vi "Read Configuration.vi"(10 "XML File Path conf":path=path "c:/ni-rt/startup/configuration.xml", 11 "Error In":errorcluster) -> (0 "Matrices":T2, 1 "Configuration":T3={"Accelerometer Bias"={"X (m/s)"=0.0, "Y (m/s)"=0.0, "Z (m/s)"=0.0}, "Gyroscope Bias"={"X (m/s)"=0.0, "Y (m/s)"=0.0, "Z (m/s)"=0.0}, "Steering Motor Gear Ratio"=611.0, "Steering Pully Gear Ratio"=1.0, "Steering Encoder CPR"=500.0, "Steering Motor Max RPM"=4000.0, "Wheelbase (m)"=1.12, "Fork Angle (rad)"=1.3, "Balancing Controller"={"Kp (/s)"=0.0, "Kd (1)"=0.0}, "Max Allowed Steering Angle (rad)"=0.7, "Task Periods"={"Emergency Stop (us)"=0, "IMU (us)"=0, "Steering Motor Encoder (us)"=0, "State Estimator (us)"=0, "Balancing Controller (us)"=0, "GNSS (us)"=0, "Logging (us)"=0, "Drive Motor (us)"=0}, "Drive Motor Gear Ratio"=0.7, "lr"=0.0, "lf"=0.0, "lambda"=0.0, "k1"=0.0, "k2"=0.0, "e1_max"=0.0, "Ad_t"=0.0, "Bd_t"=0.0, "C_t"=0.0, "D_t"=0.0, "Wheel radius"=0.311}, 2 "value":T1, 3 "Error Out":errorcluster, 5 "init trajectory 2":dbl[][](array[numeric]))   [LabVIEW 2021]
uses:
  Configuration.ctl
  <vilib>/Analysis/Matrix/Datatypes/RealMatrix.ctl
  <vilib>/Utility/xml.llb/Read From XML File(string).vi
  <vilib>/Analysis/Matrix/Numeric/Conversions/Matrix To Array - RM.vi
  <vilib>/Analysis/Matrix/NI_Matrix.lvlib
panel:
  in  "init trajectory":dbl[][](array[numeric])
  in  "XML File Path traj":path=path "c:/ni-rt/startup/trajectorylab.xml"
  in  "Init Matrix":T1
  in  "XML File Path matr":path=path "c:/ni-rt/startup/matrixlab.xml"
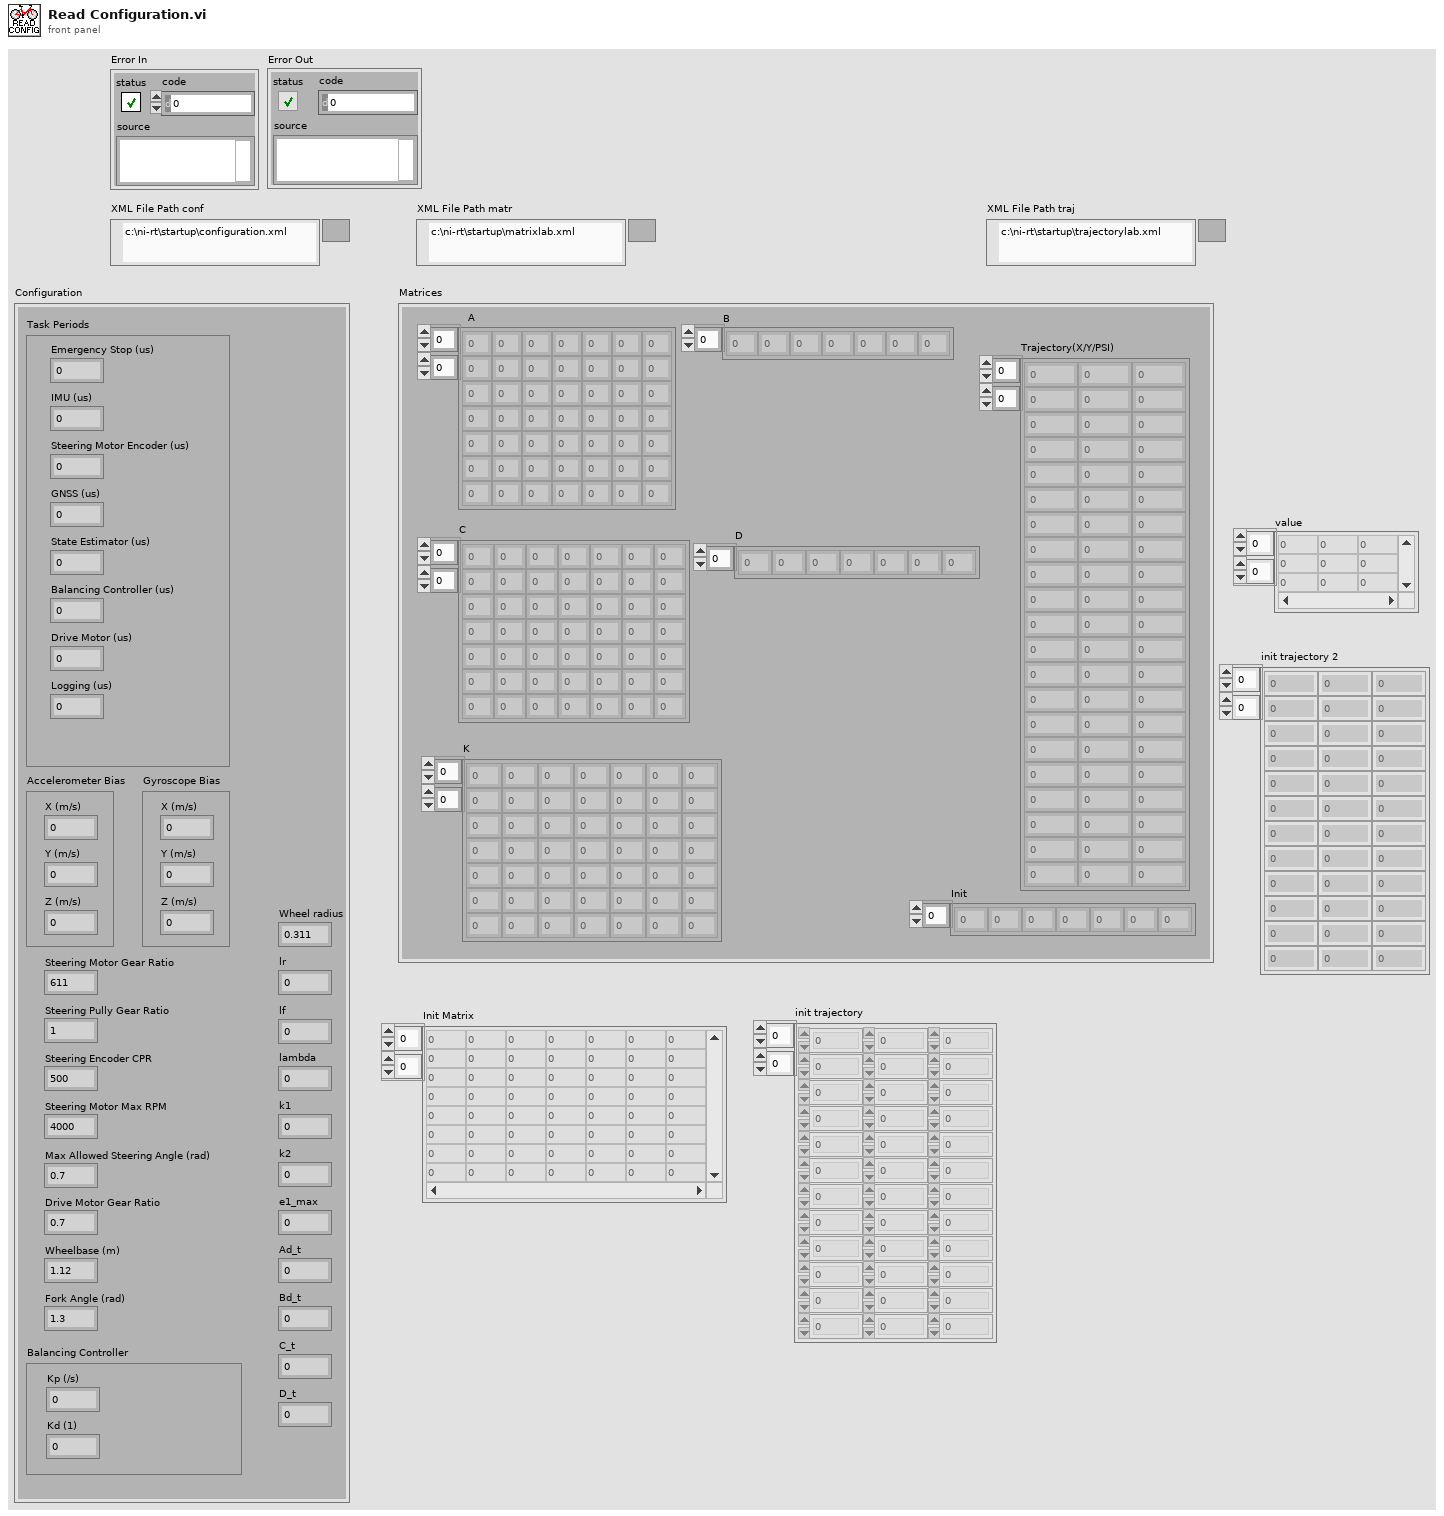
[diagram p1: front panel]
types:
  T1 = typedef "NI_Matrix.lvlib/RealMatrix.ctl" = dbl[][]
  T2 = cluster{"B":dbl[], "A":dbl[][], "C":dbl[][], "D":dbl[], "K":dbl[][], "Trajectory(X/Y/PSI)":dbl[][], "Init":dbl[]}
  T3 = typedef "Configuration.ctl" = cluster{"Accelerometer Bias":cluster{"X (m/s)":dbl, "Y (m/s)":dbl, "Z (m/s)":dbl}, "Gyroscope Bias":cluster{"X (m/s)":dbl, "Y (m/s)":dbl, "Z (m/s)":dbl}, "Steering Motor Gear Ratio":dbl, "Steering Pully Gear Ratio":dbl, "Steering Encoder CPR":dbl, "Steering Motor Max RPM":dbl, "Wheelbase (m)":dbl, "Fork Angle (rad)":dbl, "Balancing Controller":cluster{"Kp (/s)":dbl, "Kd (1)":dbl}, "Max Allowed Steering Angle (rad)":dbl, "Task Periods":cluster{"Emergency Stop (us)":i64, "IMU (us)":i64, "Steering Motor Encoder (us)":i64, "State Estimator (us)":i64, "Balancing Controller (us)":i64, "GNSS (us)":i64, "Logging (us)":i64, "Drive Motor (us)":i64}, "Drive Motor Gear Ratio":dbl, "lr":dbl, "lf":dbl, "lambda":dbl, "k1":dbl, "k2":dbl, "e1_max":dbl, "Ad_t":dbl, "Bd_t":dbl, "C_t":dbl, "D_t":dbl, "Wheel radius":dbl}
  T4 = cluster{"B":dbl[], "A":dbl[][], "C":dbl[][], "D":dbl[], "K":dbl[][], "Trajectory":dbl[][], "Init":dbl[]}
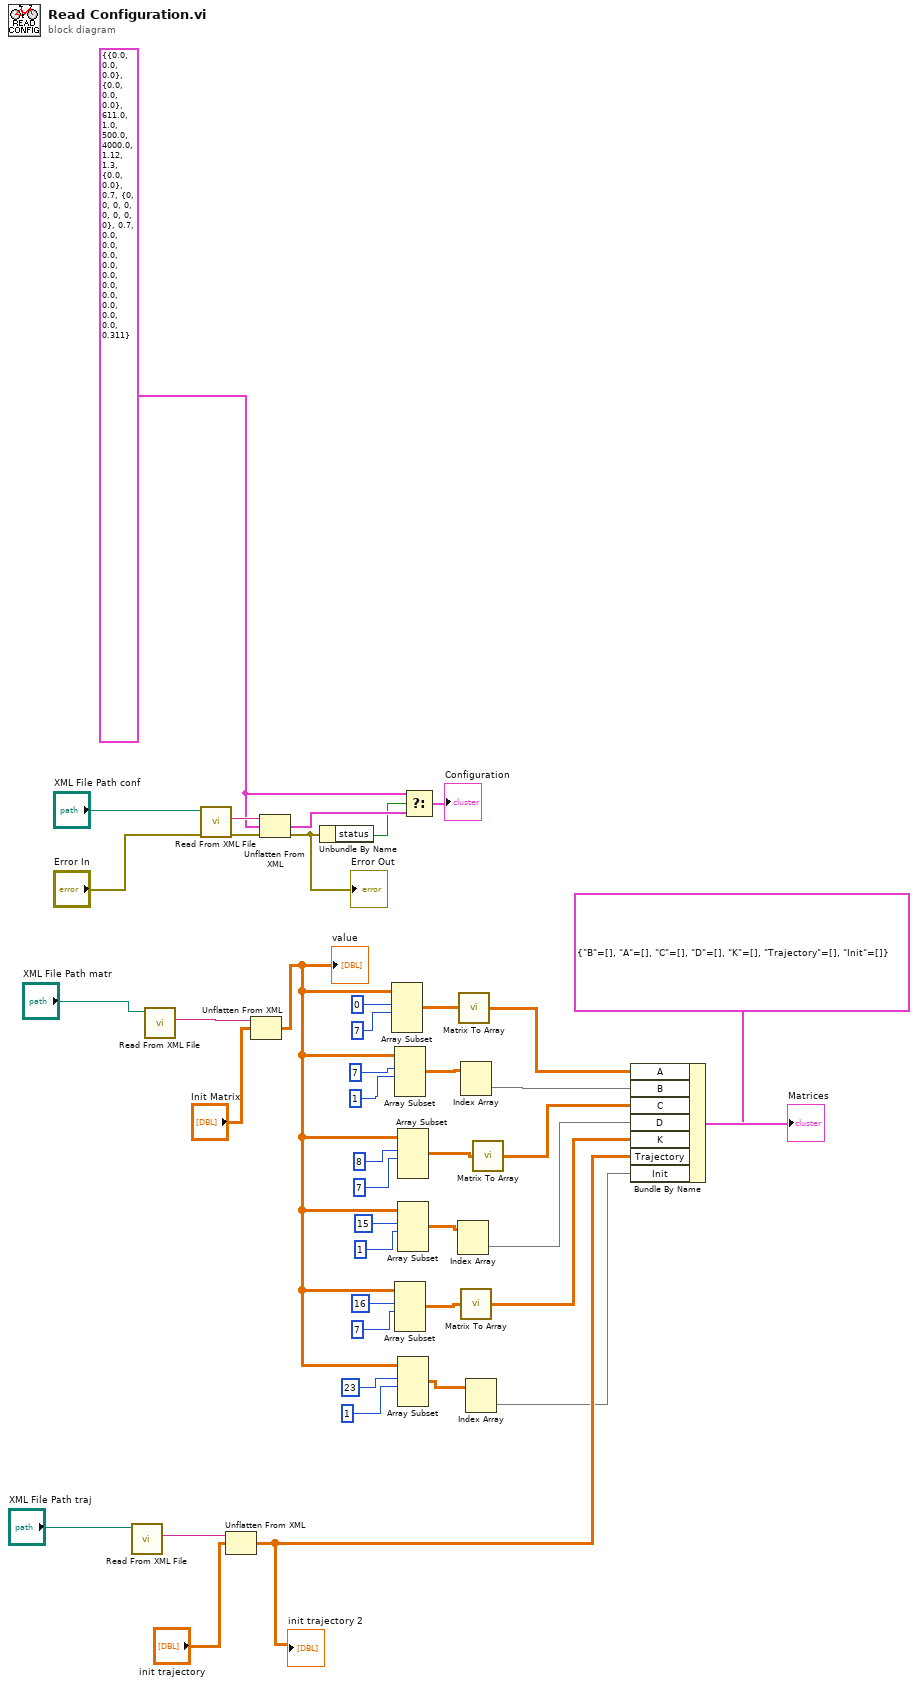
[diagram p0: block diagram]
diagram:
  w38 = T3 {"Accelerometer Bias"={"X (m/s)"=0.0, "Y (m/s)"=0.0, "Z (m/s)"=0.0}, "Gyroscope Bias"={"X (m/s)"=0.0, "Y (m/s)"=0.0, "Z (m/s)"=0.0}, "Steering Motor Gear Ratio"=611.0, "Steering Pully Gear Ratio"=1.0, "Steering Encoder CPR"=500.0, "Steering Motor Max RPM"=4000.0, "Wheelbase (m)"=1.12, "Fork Angle (rad)"=1.3, "Balancing Controller"={"Kp (/s)"=0.0, "Kd (1)"=0.0}, "Max Allowed Steering Angle (rad)"=0.7, "Task Periods"={"Emergency Stop (us)"=0, "IMU (us)"=0, "Steering Motor Encoder (us)"=0, "State Estimator (us)"=0, "Balancing Controller (us)"=0, "GNSS (us)"=0, "Logging (us)"=0, "Drive Motor (us)"=0}, "Drive Motor Gear Ratio"=0.7, "lr"=0.0, "lf"=0.0, "lambda"=0.0, "k1"=0.0, "k2"=0.0, "e1_max"=0.0, "Ad_t"=0.0, "Bd_t"=0.0, "C_t"=0.0, "D_t"=0.0, "Wheel radius"=0.311} ("Configuration")
  n1 = call-poly <vilib>:"Read From XML File.vi"("XML File Path"="XML File Path traj") -> ("XML Elements"=w9:string)  [unwired: 8 in, 2 out]
  n2 = call-poly <vilib>:"Read From XML File.vi"("XML File Path"="XML File Path matr") -> ("XML Elements"=w34:string)  [unwired: 8 in, 2 out]
  n3 = call-poly <vilib>:"Read From XML File.vi"("error in (no error)"="Error In", "XML File Path"="XML File Path conf") -> ("error out"=w43:errorcluster, "XML Elements"=w42:string)  [unwired: 7 in, 1 out]
  n4 = Unflatten From XML(xml string=w9, type="init trajectory") -> (value=w6:dbl[][])  [unwired: 1 in, 1 out]
  "init trajectory 2" <- w6
  n5 = Unflatten From XML(xml string=w34, type="Init Matrix") -> (value=w3:T1)  [unwired: 1 in, 1 out]
  "value" <- w3
  n6 = Unflatten From XML(xml string=w42, type=w38, error in (no error)=w43) -> (value=w37:T3, error out=w39:errorcluster)
  "Error Out" <- w39
  n7 = Unbundle By Name(w39) -> ("status"=w33:bool)
  n8 = Array Subset(array=w3, index (row)=0, length (row)=7) -> (w30:T1)  [unwired: 2 in]
  n9 = Array Subset(array=w3, index (row)=7, length (row)=1) -> (w16:T1)  [unwired: 2 in]
  n10 = Array Subset(array=w3, index (row)=16, length (row)=7) -> (w18:T1)  [unwired: 2 in]
  n11 = Array Subset(array=w3, index (row)=8, length (row)=7) -> (w22:T1)  [unwired: 2 in]
  n12 = Array Subset(array=w3, index (row)=15, length (row)=1) -> (w12:T1)  [unwired: 2 in]
  n13 = Array Subset(array=w3, index (row)=23, length (row)=1) -> (w2:T1)  [unwired: 2 in]
  n14 = Select(t=w38, s=w33, f=w37) -> (s? t:f=→"Configuration":T3)
  n15 = Index Array(array=w12) -> (element=w11:dbl[])  [unwired: 2 in]
  n16 = call-poly <vilib>:"Matrix To Array.vi"("Real Matrix"=w30) -> ("Real 2D Array"=w27:dbl[][])
  n17 = Index Array(array=w16) -> (element=w13:dbl[])  [unwired: 2 in]
  n18 = call-poly <vilib>:"Matrix To Array.vi"("Real Matrix"=w18) -> ("Real 2D Array"=w17:dbl[][])
  n19 = Index Array(array=w2) -> (element=w1:dbl[])  [unwired: 2 in]
  n20 = call-poly <vilib>:"Matrix To Array.vi"("Real Matrix"=w22) -> ("Real 2D Array"=w21:dbl[][])
  n21 = Bundle By Name(cluster=T4 {"B"=[], "A"=[], "C"=[], "D"=[], "K"=[], "Trajectory"=[], "Init"=[]}, "A"=w27, "B"=w13, "C"=w21, "D"=w11, "K"=w17, "Trajectory"=w6, "Init"=w1) -> (→"Matrices":T4)
